vi "Get Model From Serial Number.vi"(11 "Serial number":string) -> (3 "Model":string)   [LabVIEW 2025, in "MES Interlcok.lvlib"]
uses:
  MES Interlcok.lvlib
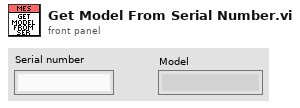
[diagram p1: front panel]
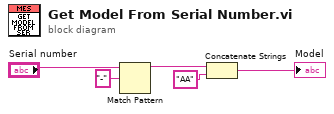
[diagram p0: block diagram]
diagram:
  n1 = Match Pattern(string="Serial number", regular expression="-") -> (before substring=w3:string)  [unwired: 1 in, 3 out]
  n2 = Concatenate Strings(w3, "AA" ("string")) -> (→"Model":string)
